vi "FPGA Image Recording (Host).vi"() -> ()   [LabVIEW 2013]
doc: "This is the host VI for the 10-Tap 8-Bit Camera with DRAM example. This example demonstrates how to acquire images from a 10-tap, 8-bit, extended configuration, Camera Link camera and display the images on the host. This example supports area scan and line scan cameras for both continuous and finite acquisitions.\n\nThis example also demonstrates the use of DRAM as a frame buffer for very high speed acquisitions. Data packing and flow-control are also employed to maximize use of the available DRAM and FIFOs in terms of both memory space and performance.\n\nAdditionally, the example demonstrates the serial server, which allows third-party camera configuration utilities to communicate with the camera using the Camera Link serial interface while this VI is running."
uses:
  <vilib>/userdefined/High Color/nirio_resource_hc.ctl
  <vilib>/rvi/interface/common/niFpgaWaitOnOcc.vi
  <vilib>/FPGAPlugInAG/PCIe-1473R/niLvFpga_Open_PCIe-1473R.vi
  <vilib>/rvi/interface/common/dynamic/niFpgaDynamicAddResources.vi
  <vilib>/FPGAPlugInAG/Dynamic/niLvFpga_Reset_Dynamic.vi
  <vilib>/Utility/error.llb/Error Cluster From Error Code.vi
  <vilib>/rvi/errors/niLvFpgaAdjustHostInterfaceError.vi
  <vilib>/FPGAPlugInAG/Dynamic/niLvFpga_Run_Dynamic.vi
  <vilib>/FPGAPlugInAG/Dynamic/niLvFpga_Close_Dynamic.vi
  <vilib>/rvi/interface/nirviOpenFPGA/nirviOpenFPGA.xnode
  LabVIEW/Vision/Vision-RIO/Vision-RIO/10-Tap 8-bit Camera with DRAM/FPGA Bitfiles/10-Tap8-bitwith_DRAM.lvbitx
  <vilib>/rvi/interface/nirviMethod/nirviMethod.xnode
  <vilib>/rvi/interface/nirviReadWriteControl/nirviReadWriteControl.xnode
  <vilib>/rvi/interface/nirviCloseFPGA/nirviCloseFPGA.xnode
  <vilib>/rvi/interface/Simulation/niFpgaSimulationCallBeginRW.vi
  <vilib>/rvi/errors/niLvFpgaMergeErrorWithErrorCode.vi
  NiFpgaLv.dll
  <vilib>/FPGAPlugInAG/Dynamic/niLvFpga_ConfigureFifo_Dynamic.vi
  <vilib>/FPGAPlugInAG/Dynamic/niLvFpga_StartFifo_Dynamic.vi
  <vilib>/FPGAPlugInAG/Dynamic/niLvFpga_ReadFifo_Dynamic.vi
panel:
  out "# of lost frames":u32
  in  "Record?":bool
  out "Codec Chosen":string="Motion JPEG (NI Vision)"
  in  "Codec index":i32=4
  out "Installed Codecs":string[](array[string])=["Microsoft Video 1", "Intel IYUV codec", "Cinepak Codec by Radius", "FF Video Codec 1 (FFV1) (NI Vision)", "Motion JPEG (NI Vision)", "Y800 Uncompressed Grey Scale (NI Vision)", "YUV 4:2:0 Planar (NI Vision)"]
  out "AVI Path":path=path "F:/Live_Data/20130925_saveFPGAframes/20130925_saveFPGAframes_test1/20130925_saveFPGAframes_test5JPEG5fps.avi"
  in  "AVI fps":u32=5
  in  "DMA Buffer Size\n(In Images)":u32=64 caption="DMA Buffer Size"
  in  "Signal Mapping":T1(ring)=enum."Basler 10-tap"
  out "Acq In Progress":bool=TRUE
  in  "Line Scan":bool
  in  "Frames To Acquire":u32 caption="Frames To Acquire\n(0 = infinite)"
  in  "Cancel":bool
  out "Acq'd Frame Width":u32=2040
  in  "Stopped":bool=TRUE
  in  "RIO Device":T2="RIO0"
  out "DMA Write Timeout":bool
  in  "Start Serial Server":bool=TRUE
  out "Frames Acq'd":u32=49
  out "Acq'd Frame Height":u32=1088
  out "Image":T3(plugin-control)
  in  "Acquire":bool
  in  "Stop":bool
  in  "Image Height":u32=1088 max=65535
  in  "Image Width":u32=2040 max=65535 step=40
  out "Initialized":bool
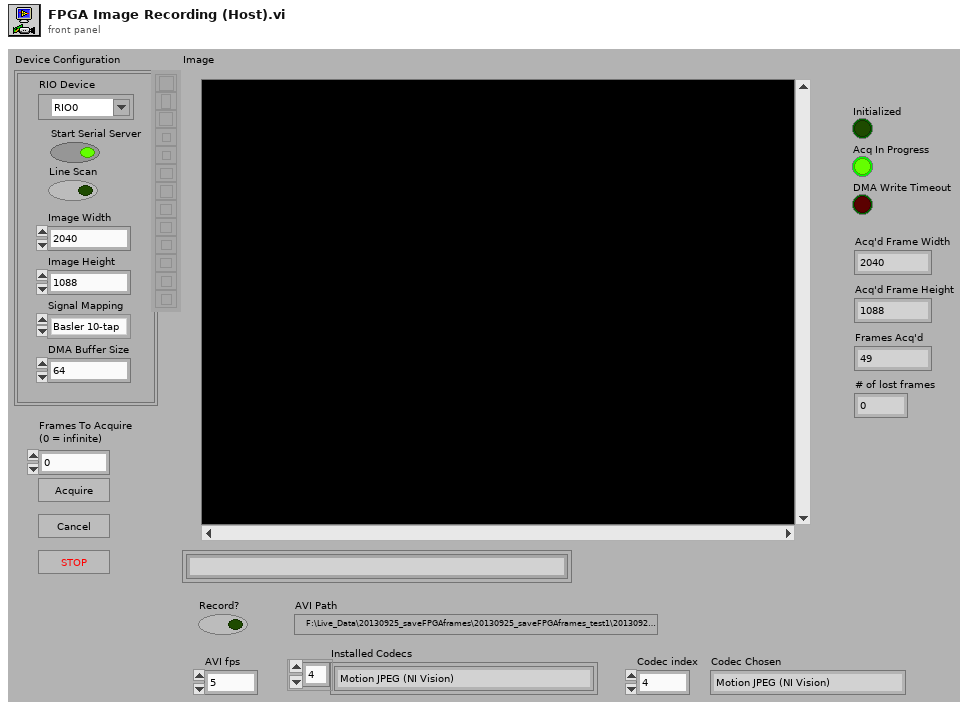
[diagram p1: front panel]
types:
  T1 = enum8{"Standard", "Basler 10-tap", "Vosskühler 10-tap"}
  T2 = typedef "nirio_resource_hc.ctl" = tag
  T3 = typedef "IMAQ Image.ctl" = refnum<image>
  T4 = typedef "Image Type" = u32
  T5 = typedef "IMAQ AVI2 Refnum.ctl" = refnum<k20>
  T6 = enum16{"big-endian, network order", "native, host order", "little-endian"}
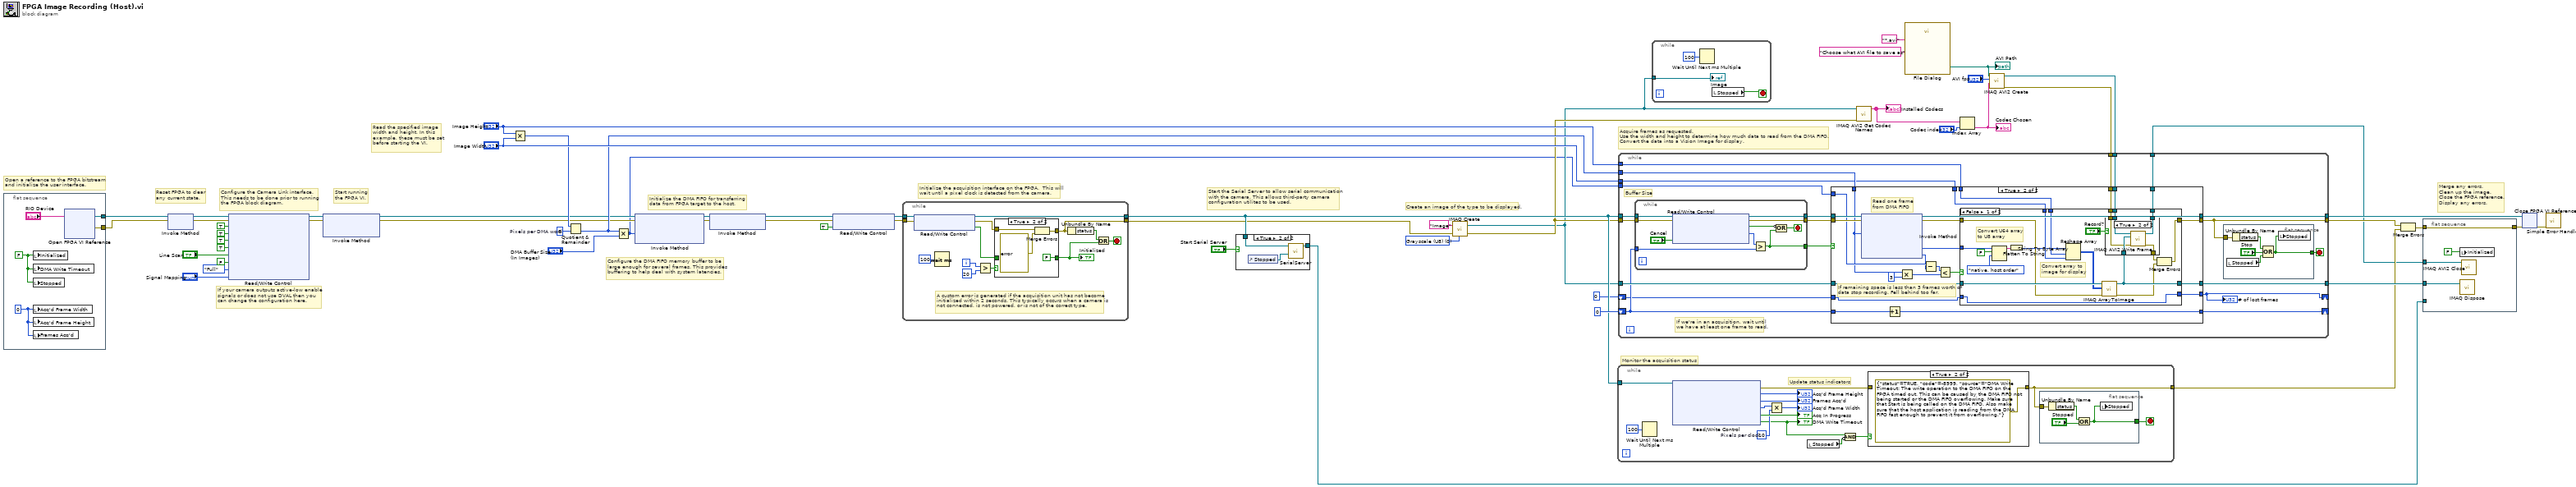
[diagram p0: block diagram]
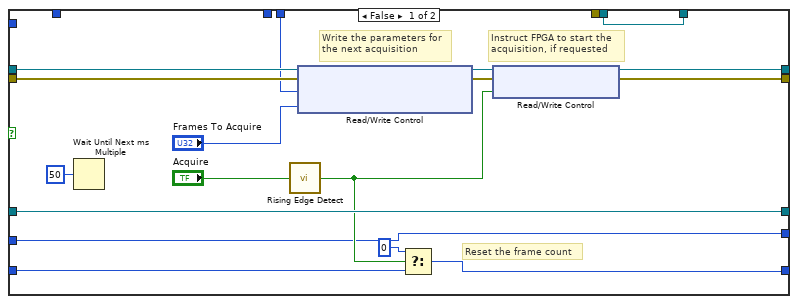
[diagram p4: hidden frame]
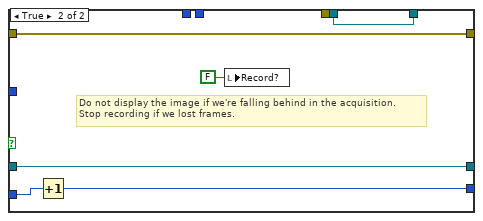
[diagram p6: hidden frame]
diagram:
  w19 = u32 8  # Pixels per DMA word
  w53 = T4 0 items=["Grayscale (U8)", "Grayscale (I16)", "Grayscale (SGL)", "Complex (CSG)", "RGB (U32)", "HSL (U32)", "RGB (U64)", "Grayscale (U16)"] ("Image Type")
  # "If your camera outputs active-low enable\nsignals or does not use DVAL then you \ncan change the configuration here."
  # "Configure the DMA FIFO memory buffer to be\nlarge enough for several frames. This provides\nbuffering to help deal with system latencies."
  # "Start running\nthe FPGA VI."
  # "Reset FPGA to clear\nany current state."
  # "Read the specified image\nwidth and height. In this\nexample, these must be set\nbefore starting the VI."
  # "Merge any errors.\nClean up the image.\nClose the FPGA reference.\nDisplay any errors."
  # "Acquire frames as requested.\nUse the width and height to determine how much data to read from the DMA FIFO.\nConvert the data into a Vision Image for display."
  # "Monitor the acquisition status"
  # "Start the Serial Server to allow serial communication\nwith the camera. This allows third-party camera\nconfiguration utilites to be used."
  # "Create an image of the type to be displayed."
  # "Initialize the acquisition interface on the FPGA.  This will\nwait until a pixel clock is detected from the camera."
  # "Initialize the DMA FIFO for transferring\ndata from FPGA target to the host."
  # "Configure the Camera Link interface.\nThis needs to be done prior to running\nthe FPGA block diagram."
  # "Open a reference to the FPGA bitstream\nand initialize the user interface."
  n1 = flat-sequence {
    tunnel: [w59] -> w44
    tunnel: [w58] -> w57
    frame #0 {
      w62 = u32 0 ("Num Lines Acq'd")
      w61 = FALSE ("stop")
      n2 = local write "Initialized"(w61) -> ()
      n3 = local write "DMA Write Timeout"(w61) -> ()
      n4 = local write "Stopped"(w61) -> ()
      n5 = local write "Acq'd Frame Width"(w62) -> ()
      n6 = local write "Acq'd Frame Height"(w62) -> ()
      n7 = local write "Frames Acq'd"(w62) -> ()
      n8 = xnode "Open FPGA VI Reference"("resource name"="RIO Device") -> ("FPGA VI Reference Out"=w59:refnum<k20>, "error out"=w58:errorcluster)  [unwired: 1 in]
    }
  }
  n9 = xnode "Invoke Method"("FPGA VI Reference In"=w44, "error in"=w57) -> ("FPGA VI Reference Out"=w33:refnum<k20>, "error out"=w36:errorcluster)
  n10 = xnode "Read/Write Control"("FPGA VI Reference In"=w33, "error in"=w36, "CL Config.FVAL Active High"=TRUE ("IO Module Config.CL FVAL Active High"), "CL Config.LVAL Active High"=TRUE ("IO Module Config.CL LVAL Active High"), "CL Config.DVAL Active High"=TRUE ("IO Module Config.CL DVAL Active High"), "CL Config.Spare Active High"=TRUE ("IO Module Config.CL Spare Active High"), "CL Config.Line Scan"="Line Scan", "Acq Control.Ignore DVAL"=FALSE ("CL Config.Line Scan"), "CL Config.Configuration"=enum8{"Base", "Medium", "Full"}."Full", "CL Config.Signal Mapping"="Signal Mapping") -> ("FPGA VI Reference Out"=w37:refnum<k20>, "error out"=w35:errorcluster)
  n11 = xnode "Invoke Method"("FPGA VI Reference In"=w37, "error in"=w35) -> ("FPGA VI Reference Out"=w16:refnum<k20>, "error out"=w15:errorcluster)  [unwired: 1 in]
  n12 = Multiply(x="Image Height", y="Image Width") -> (x*y=w18:u32)
  n13 = Quotient & Remainder(x=w18, y=w19) -> (floor(x/y)=w17:u32)  [unwired: 1 out]
  n14 = Multiply(x=w17, y="DMA Buffer Size\n(In Images)") -> (x*y=w1:u32)
  n15 = xnode "Invoke Method"("FPGA VI Reference In"=w16, "error in"=w15, "Requested Depth"=w1) -> ("FPGA VI Reference Out"=w43:refnum<k20>, "error out"=w42:errorcluster)  [unwired: 1 out]
  n16 = xnode "Invoke Method"("FPGA VI Reference In"=w43, "error in"=w42) -> ("FPGA VI Reference Out"=w28:refnum<k20>, "error out"=w41:errorcluster)
  n17 = xnode "Read/Write Control"("FPGA VI Reference In"=w28, "error in"=w41, "Acq Control.Initialize"=TRUE ("Arm Acquisition")) -> ("FPGA VI Reference Out"=w56:refnum<k20>, "error out"=w55:errorcluster)
  n18 = while {
    tunnel: w56 -> [w70]
    tunnel: w55 -> [w69]
    tunnel: [w68] -> w25
    tunnel: [w72] -> w24
    i -> [w64]
    stop <- w75 stop-if-true
    # "A custom error is generated if the acquisition unit has not become\ninitialized within 2 seconds. This typically occurs when a camera is\nnot connected, is not powered, or is not of the correct type."
    n19 = xnode "Read/Write Control"("FPGA VI Reference In"=w70, "error in"=w69) -> ("FPGA VI Reference Out"=w68:refnum<k20>, "error out"=w67:errorcluster, "Acq Status.Initialized"=w66:bool)
    n20 = Wait (ms)(milliseconds to wait=u32 100) -> ()  [unwired: 1 out]
    n21 = Greater?(x=w64, y=20) -> (0:w65:bool)
    n22 = case shown="True" w65 {
      tunnel: [w77 FALSE] -> w71
      tunnel: w66 -> [w77 _]
      tunnel: w67 -> [w76 w79]
      tunnel: [w76 w81] -> w72
      frame False {
      }
      frame True {
        n23 = Merge Errors(w79, errorcluster {"status"=TRUE, "code"=-8999, "source"="Acquisition Initialization: This error typically occurs when a camera is not properly connected, is not powered, or is not of the correct type."} ("error in")) -> (w81:errorcluster)
      }
    }
    "Initialized" <- w71
    n24 = Unbundle By Name(w72) -> ("status"=w74:bool)
    n25 = Or(x=w74, y=w71) -> (x .or. y?=w75:bool)
  }
  n26 = case shown="True" "Start Serial Server" {
    tunnel: [_ w82] -> w45
    tunnel: w25 -> [_ w83]
    frame False {
    }
    frame True {
      n27 = control-ref of="Stopped"() -> (w84:refnum<vi>)
      n28 = call "SerialServer.vi"("Stop Refnum"=w84, "FPGA VI Reference In"=w83) -> ("FPGA VI Reference Out"=w82:refnum<k20>)  [unwired: 5 in]
    }
  }
  n29 = call "IMAQ Create"("Image Name"="Image", "Image Type"=w53, "error in (no error)"=w24) -> ("New Image"=w2:T3, "error out"=w4:errorcluster)  [unwired: 2 in]
  n30 = while {
    tunnel: w25 -> [w95]
    tunnel: [w98] -> w38
    stop <- w97 stop-if-true
    w88 = u32 10  # Pixels per clock
    # "Update status indicators"
    n31 = Wait Until Next ms Multiple(millisecond multiple=u32 100) -> ()  [unwired: 1 out]
    n32 = xnode "Read/Write Control"("FPGA VI Reference In"=w95) -> ("error out"=w94:errorcluster, "Acq Status.Lines Per Frame"=→"Acq'd Frame Height":u32, "Acq Status.Frames Acq'd"=→"Frames Acq'd":u32, "Acq Status.Clocks Per Line"=w89:u32, "Acq Status.Acq In Progress"=→"Acq In Progress":bool, "Acq Status.DMA Write Timeout"=w86:bool)  [unwired: 1 in, 1 out]
    "DMA Write Timeout" <- w86
    n33 = Multiply(x=w89, y=w88) -> (x*y=→"Acq'd Frame Width":u32)
    n34 = local read "Stopped"() -> (w85:bool)
    n35 = Compound Arithmetic op=AND(w86, invert w85) -> (w87:bool)
    n36 = case shown="True" w87 {
      tunnel: w94 -> [w103 _]
      tunnel: [w103 errorcluster {"status"=TRUE, "code"=-8999, "source"="DMA Write Timeout: The write operation to the DMA FIFO on the FPGA timed out. This can be caused by the DMA FIFO not being started or the DMA FIFO overflowing. Make sure that Start is being called on the DMA FIFO. Also make sure that the host application is reading from the DMA FIFO fast enough to prevent it from overflowing."} ("error out")] -> w98
      frame False {
      }
      frame True {
      }
    }
    n37 = flat-sequence {
      tunnel: w98 -> [w102]
      tunnel: [w100] -> w97
      frame #0 {
        n38 = Unbundle By Name(w102) -> ("status"=w101:bool)
        n39 = Or(x=w101, y="Stopped") -> (x .or. y?=w100:bool)
        n40 = local write "Stopped"(w100) -> ()
      }
    }
  }
  n41 = while {
    tunnel: w2 -> [w107]
    stop <- w105 stop-if-true
    n42 = Wait Until Next ms Multiple(millisecond multiple=u32 100) -> ()  [unwired: 1 out]
    n43 = local read "Stopped"() -> (w105:bool)
    "Image" <- w107
  }
  n44 = call "IMAQ AVI2 Get Codec Names"("error in (no error)"=w4, "Image"=w2) -> ("Codec Names"=w8:string[])  [unwired: 8 in, 1 out]
  "Installed Codecs" <- w8
  n45 = call "File Dialog"("prompt"="Choose what AVI file to save as", "pattern (all files)"="*.avi" ("pattern label")) -> ("selected path"=w11:path)  [unwired: 10 in, 3 out]
  "AVI Path" <- w11
  n46 = Index Array(array=w8, index="Codec index") -> (element=w12:string)
  "Codec Chosen" <- w12
  n47 = call "IMAQ AVI2 Create"("Codec"=w12, "Frames Per Second"="AVI fps", "AVI Path"=w11) -> ("error out"=w6:errorcluster, "AVI Refnum"=w7:T5)  [unwired: 7 in]
  n48 = while {
    tunnel: w25 -> [w120]
    tunnel: w4 -> [w119]
    tunnel: w17 -> [w128]
    tunnel: "Image Height" -> [w127]
    tunnel: "Image Width" -> [w126]
    tunnel: w2 -> [w125]
    tunnel: [w123] -> w39
    tunnel: [w124] -> w52
    tunnel: [w121] -> w47
    shift-right: [w115] -> _
    shift-left: u32 0 -> [w114]
    tunnel: w7 -> [w113]
    tunnel: w6 -> [w112]
    tunnel: [w111] -> w14
    shift-right: [w110] -> _
    shift-left: u32 0 -> [w109]
    tunnel: w1 -> [w108]
    stop <- w122 stop-if-true
    # "Buffer Size"
    # "If we're in an acquisition, wait until\nwe have at least one frame to read."
    n49 = while {
      tunnel: w120 -> [w135]
      tunnel: w119 -> [w134]
      tunnel: [w132] -> w118
      tunnel: [w133] -> w117
      tunnel: w114 -> [w138]
      tunnel: [w136] -> w116
      stop <- w137 stop-if-true
      n50 = xnode "Read/Write Control"("FPGA VI Reference In"=w135, "error in"=w134, "Acq Control.Cancel Acq"="Cancel") -> ("FPGA VI Reference Out"=w133:refnum<k20>, "error out"=w132:errorcluster, "Acq Status.Acq In Progress"=w131:bool, "Acq Status.Frames Acq'd"=w130:u32)
      n51 = Greater?(x=w130, y=w138) -> (0:w136:bool)
      n52 = Compound Arithmetic op=OR(invert w131, w136) -> (w137:bool)
    }
    n53 = case shown="True" w116 {
      tunnel: w117 -> [w156 w177]
      tunnel: w118 -> [w155 w176]
      tunnel: w128 -> [_ w164]
      tunnel: w127 -> [w149 w184]
      tunnel: w126 -> [_ w183]
      tunnel: w125 -> [w160 w182]
      tunnel: [w151 w180] -> w123
      tunnel: [w154 w179] -> w124
      tunnel: [w160 w178] -> w121
      tunnel: w114 -> [w157 w175]
      tunnel: [w159 w174] -> w115
      tunnel: w113 -> [w145 w171]
      tunnel: w112 -> [_ w170]
      tunnel: [w145 w169] -> w111
      tunnel: [w144 w168] -> w110
      tunnel: w109 -> [w144 w167]
      tunnel: w108 -> [_ w166]
      frame False {
        # "Reset the frame count"
        # "Instruct FPGA to start the\nacquisition, if requested"
        # "Write the parameters for\nthe next acquisition"
        n54 = Wait Until Next ms Multiple(millisecond multiple=u32 50) -> ()  [unwired: 1 out]
        n55 = call "Rising Edge Detect.vi"("Input"="Acquire") -> ("Pulse"=w146:bool)  [unwired: 4 in]
        n56 = xnode "Read/Write Control"("FPGA VI Reference In"=w156, "error in"=w155, "Acq Control.Line Scan Height"=w149, "Acq Control.Frames To Acq"="Frames To Acquire") -> ("FPGA VI Reference Out"=w153:refnum<k20>, "error out"=w152:errorcluster)
        n57 = Select(t=u32 0, s=w146, f=w157) -> (s? t:f=w159:u32)
        n58 = xnode "Read/Write Control"("FPGA VI Reference In"=w153, "error in"=w152, "Acq Control.Acquire"=w146) -> ("FPGA VI Reference Out"=w154:refnum<k20>, "error out"=w151:errorcluster)
      }
      frame True {
        # "If remaining space is less than 3 frames worth of data stop recording. Fell behind too far."
        # "Read one frame\nfrom DMA FIFO"
        n59 = xnode "Invoke Method"("FPGA VI Reference In"=w177, "error in"=w176, "Number of Elements"=w164) -> ("FPGA VI Reference Out"=w179:refnum<k20>, "error out"=w181:errorcluster, "Data"=w173:u64[], "Elements Remaining"=w165:u32)  [unwired: 1 in]
        n60 = Increment(x=w175) -> (x+1=w174:u32)
        n61 = Multiply(x=w164, y=u32 3) -> (x*y=w162:u32)
        n62 = Subtract(x=w166, y=w165) -> (x-y=w161:u32)
        n63 = Less?(x=w161, y=w162) -> (x < y?=w172:bool)
        n64 = case shown="False" w172 {
          tunnel: w184 -> [w203 _]
          tunnel: w183 -> [w202 _]
          tunnel: w182 -> [w201 w216]
          tunnel: w181 -> [w200 w215]
          tunnel: [w187 w215] -> w180
          tunnel: [w192 w216] -> w178
          tunnel: w173 -> [w197 _]
          tunnel: w171 -> [w193 w214]
          tunnel: w170 -> [w191 _]
          tunnel: [w190 w214] -> w169
          tunnel: [w185 w213] -> w168
          tunnel: w167 -> [w185 w212]
          frame False {
            # "Convert U64 array\nto U8 array"
            # "Convert array to\nimage for display"
            n65 = Flatten To String(anything=w197, prepend array or string size? (T)=FALSE, byte order (0:big-endian, network order)=T6."native, host order") -> (data string=w195:string)  [unwired: 1 in, 2 out]
            n66 = String To Byte Array(string=w195) -> (unsigned byte array=w194:u8[])
            n67 = Reshape Array(w194, w203, w202) -> (w199:u8[][])
            n68 = call "IMAQ ArrayToImage"("error in (no error)"=w200, "Image Pixels (U8)"=w199, "Image"=w201) -> ("error out"=w188:errorcluster, "Image Out"=w192:T3)  [unwired: 7 in]
            n69 = case shown="True" "Record?" {
              tunnel: w193 -> [w204 w210]
              tunnel: w192 -> [_ w209]
              tunnel: w191 -> [w205 w208]
              tunnel: [w204 w207] -> w190
              tunnel: [w205 w206] -> w189
              frame False {
              }
              frame True {
                n70 = call "IMAQ AVI2 Write Frame"("error in (no error)"=w208, "Image"=w209, "AVI Refnum"=w210) -> ("error out"=w206:errorcluster, "AVI Refnum (duplicate)"=w207:T5)  [unwired: 6 in, 1 out]
              }
            }
            n71 = Merge Errors(w189, w188) -> (w187:errorcluster)
          }
          frame True {
            # "Do not display the image if we're falling behind in the acquisition.\nStop recording if we lost frames."
            n72 = Increment(x=w212) -> (x+1=w213:u32)
            n73 = local write "Record?"(FALSE ("Record?")) -> ()
          }
        }
      }
    }
    "# of lost frames" <- w110
    n74 = flat-sequence {
      tunnel: w123 -> [w141]
      tunnel: [w140] -> w122
      frame #0 {
        n75 = local read "Stopped"() -> (w139:bool)
        n76 = Unbundle By Name(w141) -> ("status"=w142:bool)
        n77 = Compound Arithmetic op=OR(w142, "Stop", w139) -> (w140:bool)
        n78 = local write "Stopped"(w140) -> ()
      }
    }
  }
  n79 = Merge Errors(w39, w38) -> (w40:errorcluster)
  n80 = flat-sequence {
    tunnel: w40 -> [w219]
    tunnel: [w219] -> w49
    tunnel: w47 -> [w220]
    tunnel: w45 -> [_]
    tunnel: w14 -> [w217]
    frame #0 {
      n81 = local write "Initialized"(FALSE ("Module Enabled")) -> ()
      n82 = call "IMAQ Dispose"("Image"=w220) -> ()  [unwired: 5 in, 1 out]
      n83 = call "IMAQ AVI2 Close"("AVI Refnum"=w217) -> ()  [unwired: 10 in, 1 out]
    }
  }
  n84 = xnode "Close FPGA VI Reference"("FPGA VI Reference In"=w52, "error in"=w49) -> ("error out"=w46:errorcluster)
  n85 = call <vilib>:"Simple Error Handler.vi"("error in (no error)"=w46) -> ()  [unwired: 4 in, 5 out]
